vi "PantherLAB_Log - Create New DQMH Event.vi"(9 "Ephemeral Scripting Info":T1, 10 "Event Info":T2 {"timeout (ms)" min=-1 step=1}, 11 "Module Info":T5) -> (0 "error out":errorcluster)   [LabVIEW 2016]
doc: "_____\nCreated using DQMH Framework: Event Scripter 7.1.0.1450."
uses:
  <vilib>/Delacor/Delacor QMH/Libraries/_Scripting Support/Module Info--cluster.ctl
  <vilib>/Delacor/Delacor QMH/Libraries/_Scripting Support/Module Type--enum.ctl
  <vilib>/Delacor/Delacor QMH/Libraries/_Scripting Support/Event Info (New)--cluster.ctl
  <vilib>/Delacor/Delacor QMH/Libraries/_Scripting Support/Event Type (New)--enum.ctl
  <vilib>/Delacor/Delacor QMH/Libraries/_Scripting Support/Request Scoping--enum.ctl
  <vilib>/Delacor/Delacor QMH/Libraries/_Scripting Support/Ephemeral Scripting Info--cluster.ctl
  <resource>/dialog/lvconfig.llb/LV Config Read Boolean.vi
  PantherLAB Scripting Hooks/PantherLAB_Scripting.lvlib
  <vilib>/Delacor/Delacor QMH/Libraries/_Scripting Support/dqmh_lib_DQMH Scripting Support.lvlib
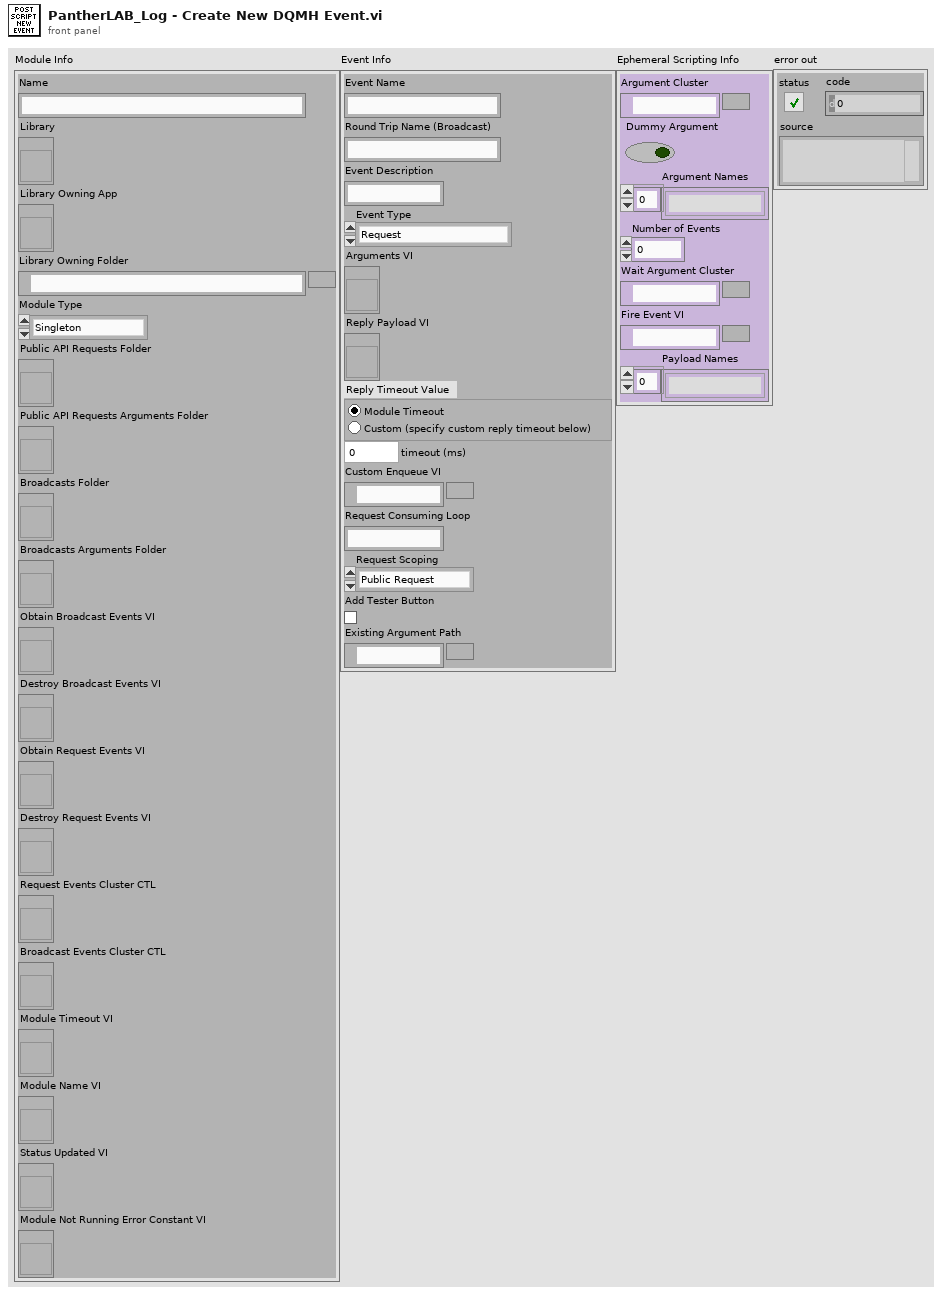
[diagram p1: front panel]
types:
  T1 = typedef "dqmh_lib_DQMH Scripting Support.lvlib/Ephemeral Scripting Info--cluster.ctl" = cluster{"Argument Cluster":path, "Dummy Argument":bool, "Argument Names":string[], "Number of Events":i32, "Wait Argument Cluster":path, "Fire Event VI":path, "Payload Names":string[]}
  T2 = typedef "dqmh_lib_DQMH Scripting Support.lvlib/Event Info (New)--cluster.ctl" = cluster{"Event Name":string, "Round Trip Name (Broadcast)":string, "Event Description":string, "Event Type":T3, "Arguments VI":refnum<vi>, "Reply Payload VI":refnum<vi>, "Reply Timeout Value":enum32{"Module Timeout", "Custom"}, "timeout (ms)":i32, "Custom Enqueue VI":path, "Request Consuming Loop":string, "Request Scoping":T4, "Add Tester Button":bool, "Existing Argument Path":path}
  T3 = typedef "dqmh_lib_DQMH Scripting Support.lvlib/Event Type (New)--enum.ctl" = enum16{"Request", "Broadcast", "Request and Wait for Reply", "Round Trip"}
  T4 = typedef "dqmh_lib_DQMH Scripting Support.lvlib/Request Scoping--enum.ctl" = enum16{"Public Request", "Private Request", "Local Instance"}
  T5 = typedef "dqmh_lib_DQMH Scripting Support.lvlib/Module Info--cluster.ctl" = cluster{"Name":string, "Library":refnum<vi>, "Library Owning App":refnum<vi>, "Library Owning Folder":path, "Module Type":T6, "Public API Requests Folder":refnum<vi>, "Public API Requests Arguments Folder":refnum<vi>, "Broadcasts Folder":refnum<vi>, "Broadcasts Arguments Folder":refnum<vi>, "Obtain Broadcast Events VI":refnum<vi>, "Destroy Broadcast Events VI":refnum<vi>, "Obtain Request Events VI":refnum<vi>, "Destroy Request Events VI":refnum<vi>, "Request Events Cluster CTL":refnum<vi>, "Broadcast Events Cluster CTL":refnum<vi>, "Module Timeout VI":refnum<vi>, "Module Name VI":refnum<vi>, "Status Updated VI":refnum<vi>, "Module Not Running Error Constant VI":refnum<vi>}
  T6 = typedef "dqmh_lib_DQMH Scripting Support.lvlib/Module Type--enum.ctl" = enum16{"Singleton", "Cloneable"}
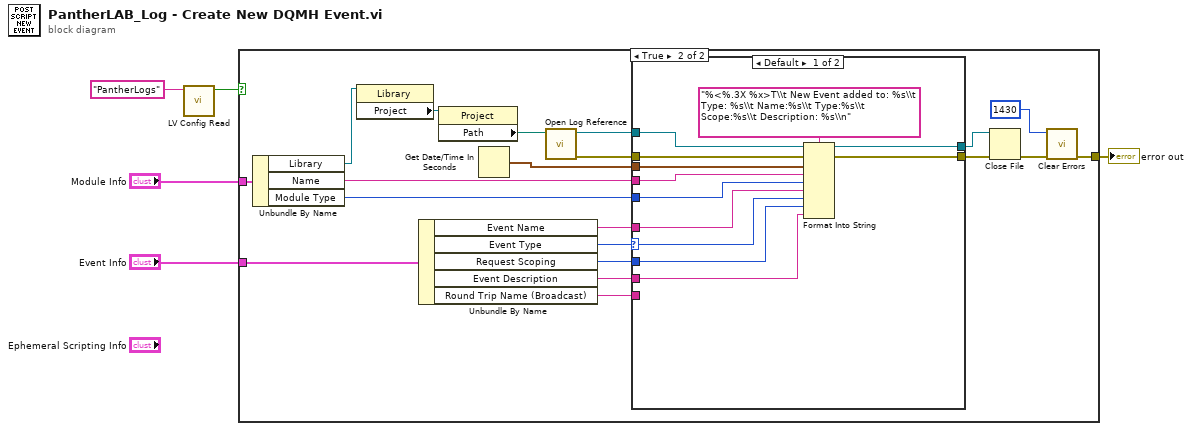
[diagram p0: block diagram]
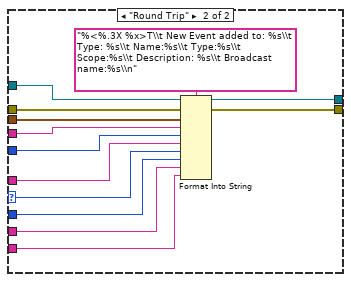
[diagram p3: hidden frame]
diagram:
  n1 = call-poly <resource>:"LV Config Read.vi"("key"="PantherLogs") -> ("value"=w1:bool)  [unwired: 4 in, 2 out]
  n2 = case shown="True" w1 {
    tunnel: [_ w7] -> w5
    tunnel: "Module Info" -> [_ w22]
    tunnel: "Event Info" -> [_ w19]
    frame False {
    }
    frame True {
      n3 = Unbundle By Name(w22) -> ("Library"=w21:refnum<vi>, "Name"=w16:string, "Module Type"=w15:T6)
      n4 = property class="Library"(reference=w21) -> ("Project"=w20:refnum<vi>)  [unwired: 1 in, 2 out]
      n5 = Unbundle By Name(w19) -> ("Event Name"=w11:string, "Event Type"=w12:T3, "Request Scoping"=w10:T4, "Event Description"=w9:string, "Round Trip Name (Broadcast)"=w8:string)
      n6 = property class="Project"(reference=w20) -> ("Path"=w13:path)  [unwired: 1 in, 2 out]
      n7 = Get Date/Time In Seconds() -> (seconds since 1Jan1904=w14:timestamp)
      n8 = call "Open Log Reference.vi"("Project Path"=w13) -> ("error out"=w25:errorcluster, "File Reference"=w18:refnum<file>)  [unwired: 9 in]
      n9 = case shown="Default" w12 {
        selector: w12 -> [w29 w42]
        tunnel: w18 -> [w35 w48]
        tunnel: w25 -> [w37 w50]
        tunnel: [w34 w47] -> w17
        tunnel: [w36 w49] -> w24
        tunnel: w16 -> [w32 w45]
        tunnel: w15 -> [w33 w46]
        tunnel: w14 -> [w31 w44]
        tunnel: w11 -> [w30 w43]
        tunnel: w10 -> [w28 w41]
        tunnel: w9 -> [w27 w40]
        tunnel: w8 -> [_ w38]
        frame Default {
          n10 = Format Into String(format string="%<%.3X %x>T\\t New Event added to: %s\\t Type: %s\\t Name:%s\\t Type:%s\\t Scope:%s\\t Description: %s\\n", initial string=w35, error in=w37, w31, w32, w33, w30, w29, w28, w27) -> (resulting string=w34:refnum<file>, error out=w36:errorcluster)
        }
        frame "Round Trip" {
          n11 = Format Into String(format string="%<%.3X %x>T\\t New Event added to: %s\\t Type: %s\\t Name:%s\\t Type:%s\\t Scope:%s\\t Description: %s\\t Broadcast name:%s\\n", initial string=w48, error in=w50, w44, w45, w46, w43, w42, w41, w40, w38) -> (resulting string=w47:refnum<file>, error out=w49:errorcluster)
        }
      }
      n12 = Close File(refnum=w17, error in=w24) -> (error out=w23:errorcluster)  [unwired: 1 out]
      n13 = call <vilib>:"Clear Errors.vi"("error in (no error)"=w23, "specific error code to clear (0: all)"=1430) -> ("error out"=w7:errorcluster)  [unwired: 4 in, 1 out]
    }
  }
  "error out" <- w5
